vi "未公开函数.vi"   [LabVIEW 2011]
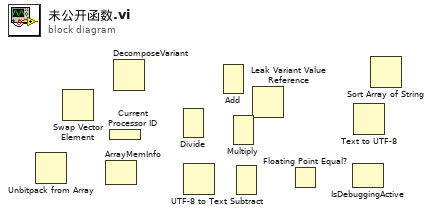
[diagram p0: block diagram]
diagram:
  n1 = Unbitpack from Array() -> ()  [unwired: 2 in, 1 out]
  n2 = Swap Vector Element() -> ()  [unwired: 3 in, 3 out]
  n3 = ArrayMemInfo() -> ()  [unwired: 7 in, 4 out]
  n4 = Current Processor ID ("当前进程ID")() -> ()  [unwired: 1 out]
  n5 = DecomposeVariant() -> ()  [unwired: 2 in, 4 out]
  n6 = Divide() -> ()  [unwired: 3 in, 2 out]
  n7 = UTF-8 to Text() -> ()  [unwired: 2 in, 2 out]
  n8 = Add() -> ()  [unwired: 3 in, 2 out]
  n9 = Multiply() -> ()  [unwired: 3 in, 2 out]
  n10 = Subtract() -> ()  [unwired: 3 in, 2 out]
  n11 = Leak Variant Value Reference() -> ()  [unwired: 2 in, 2 out]
  n12 = Floating Point Equal?() -> ()  [unwired: 3 in, 1 out]
  n13 = IsDebuggingActive() -> ()  [unwired: 10 in, 1 out]
  n14 = Text to UTF-8() -> ()  [unwired: 2 in, 2 out]
  n15 = Sort Array of String() -> ()  [unwired: 1 in, 1 out]
